vi "Init - Check Duplex.vi"(7 "Duplex Packets":refnum<data-value>, 8 "error in (no error)":errorcluster, 10 "Receive Packet ID":i32=-1, 11 "Transmit Packet ID":i32=-1) -> (0 "error out":errorcluster, 2 "Duplex Settings":T1, 3 "Is Duplex?":bool)   [LabVIEW 2021, in "UDP-Custom-Device Engine.lvlib"]
uses:
  UDP-Custom-Device Engine.lvlib
  Shared/Types/Shared - Duplex Settings.ctl
  Shared/UDP-Custom-Device Shared.lvlib
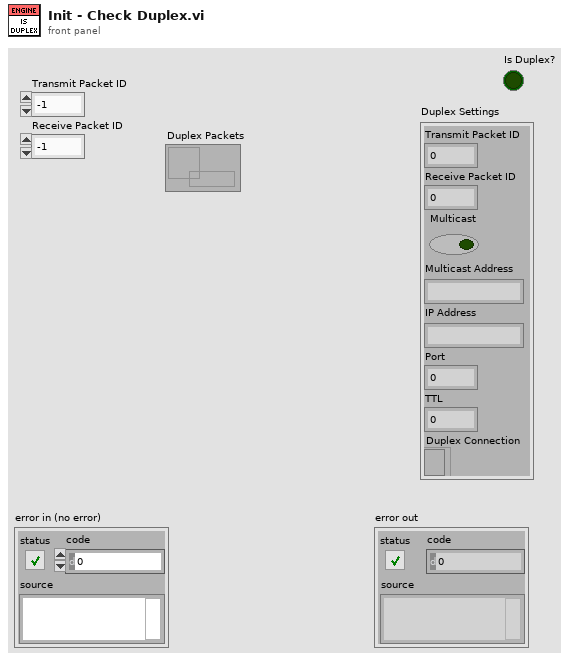
[diagram p1: front panel]
types:
  T1 = typedef "UDP-Custom-Device Shared.lvlib/Shared - Duplex Settings.ctl" = cluster{"Transmit Packet ID":i32, "Receive Packet ID":i32, "Multicast":bool, "Multicast Address":string, "IP Address":string, "Port":u16, "TTL":u16, "Duplex Connection":refnum<k16>}
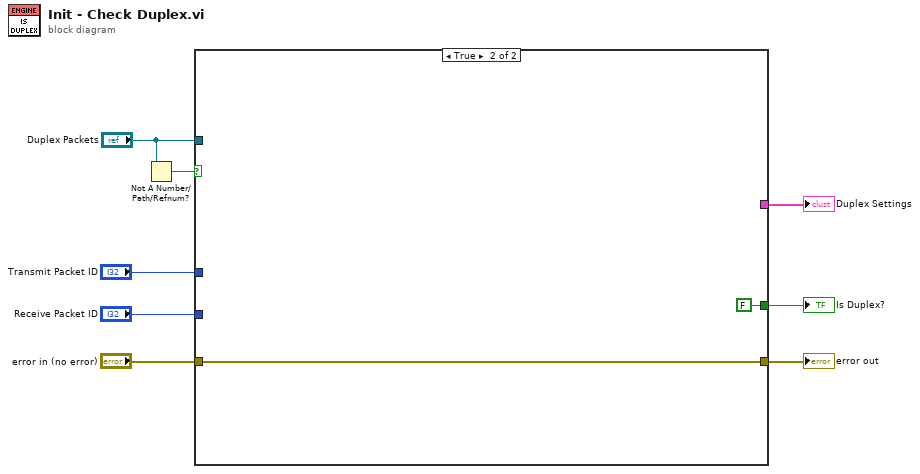
[diagram p0: block diagram]
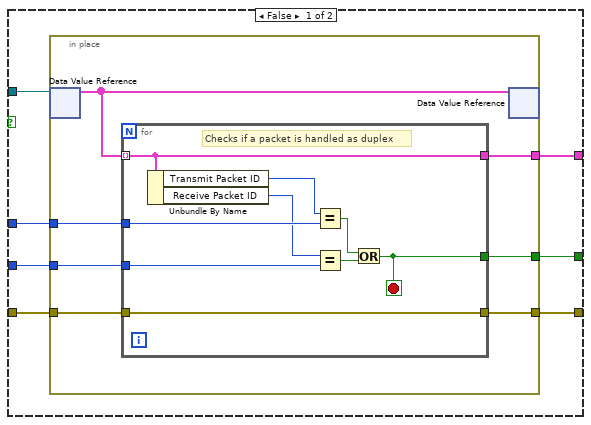
[diagram p2: hidden frame]
diagram:
  n1 = Not A Number/Path/Refnum?(number/path/refnum="Duplex Packets") -> (NaN/Path/Refnum?=w2:bool)
  n2 = case shown="True" w2 {
    tunnel: "Transmit Packet ID" -> [w15 _]
    tunnel: "Receive Packet ID" -> [w14 _]
    tunnel: "error in (no error)" -> [w13 w32]
    tunnel: [w12 w32] -> w5
    tunnel: [w11 FALSE] -> w4
    tunnel: [w10 _] -> w3
    tunnel: "Duplex Packets" -> [w9 _]
    frame False {
      n3 = in-place {
        in-place-border: w15 -> [w22]
        in-place-border: w14 -> [w21]
        in-place-border: w13 -> [w20]
        in-place-border: [w19] -> w12
        in-place-border: [w18] -> w11
        in-place-border: [w17] -> w10
        n4 = in-place-dvr #1(w9) -> (w16:T1[])  [unwired: 1 out]
        n5 = for {
          tunnel: w16 -> [w24] mode=indexing
          tunnel: w22 -> [w28]
          tunnel: w21 -> [w27]
          tunnel: w20 -> [w25]
          tunnel: [w25] -> w19
          tunnel: [w24] -> w17
          tunnel: [w23] -> w18
          stop <- w23 stop-if-true
          # "Checks if a packet is handled as duplex"
          n6 = Unbundle By Name(w24) -> ("Transmit Packet ID"=w29:i32, "Receive Packet ID"=w26:i32)
          n7 = Equal?(x=w29, y=w28) -> (x = y?=w31:bool)
          n8 = Equal?(x=w26, y=w27) -> (x = y?=w30:bool)
          n9 = Or(x=w31, y=w30) -> (x .or. y?=w23:bool)
        }
        n10 = in-place-dvr #1(w16) -> ()  [unwired: 2 out]
      }
    }
    frame True {
    }
  }
  "error out" <- w5
  "Is Duplex?" <- w4
  "Duplex Settings" <- w3
